vi "nm_string.vi"(8 "error in (no error)":errorcluster, 10 "Grating, gr/mm":u16(ring)=2 items=["2400", "1800", "1200", "600", "300", "150"], 11 "Wavelength, nm":dbl format="%.3f") -> (0 "error out":errorcluster, 3 "nm_String":string)   [LabVIEW 2017, in "Monochromator.lvlib" / "PTI.lvlib"]
doc: "convert wavelength to step"
uses:
  PTI.lvlib
panel:
  out "number of steps":i32
  # "nm"
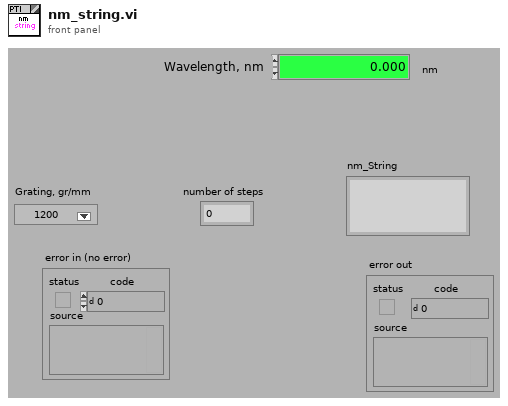
[diagram p1: front panel]
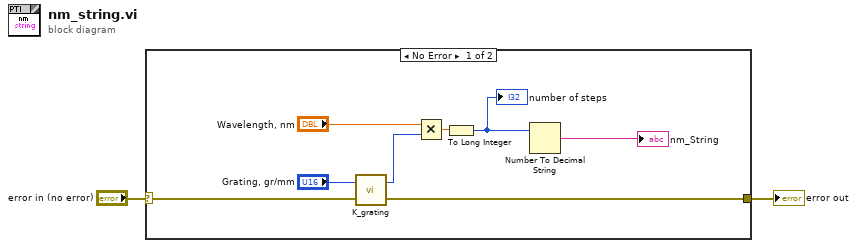
[diagram p0: block diagram]
diagram:
  n1 = case shown="No Error" "error in (no error)" {
    selector: "error in (no error)" -> [w8 w11]
    tunnel: [w9 w11] -> w1
    frame No Error {
      n2 = call "K_grating.vi"("error in (no error)"=w8, "Grating, gr/mm 2"="Grating, gr/mm") -> ("error out"=w9:errorcluster, "K_grating"=w7:i16)
      n3 = Multiply(x="Wavelength, nm", y=w7) -> (x*y=w6:dbl)
      n4 = To Long Integer(number=w6) -> (32bit integer=w5:i32)
      "number of steps" <- w5
      n5 = Number To Decimal String(number=w5) -> (decimal integer string=→"nm_String":string)  [unwired: 1 in]
    }
    frame Error {
    }
  }
  "error out" <- w1
